vi "Write Encoder Offsets Global.vi"(0 "Swerve 4":i32, 1 "Swerve 3":i32, 2 "Swerve 2":i32, 3 "Swerve 1":i32) -> ()   [LabVIEW 2016]
uses:
  Main/Robot Global Data.vi
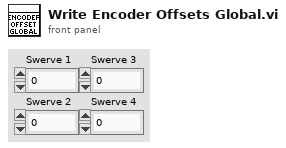
[diagram p1: front panel]
types:
  T1 = cluster{"Swerve 1":i32, "Swerve 2":i32, "Swerve 3":i32, "Swerve 4":i32}
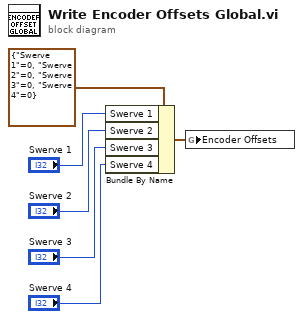
[diagram p0: block diagram]
diagram:
  n1 = Bundle By Name(cluster=T1 {"Swerve 1"=0, "Swerve 2"=0, "Swerve 3"=0, "Swerve 4"=0} ("input cluster"), "Swerve 1"="Swerve 1", "Swerve 2"="Swerve 2", "Swerve 3"="Swerve 3", "Swerve 4"="Swerve 4") -> (w5:T1)
  n2 = global write "Robot Global Data.vi" "Encoder Offsets"(w5) -> ()
